vi "Defer Panel Updates.vi"(7 "Set Defer (T)":bool=TRUE, 8 "error in (no error)":errorcluster, 9 "Front Panel (Lookup)":refnum<vi>, 10 "Defer":bool, 11 "Tree (Front Panel)":refnum<vi>) -> (0 "error out":errorcluster, 1 "Front Panel":refnum<vi>)   [LabVIEW 2026, in "Tree Map.lvlib"]
uses:
  Tree Map.lvlib
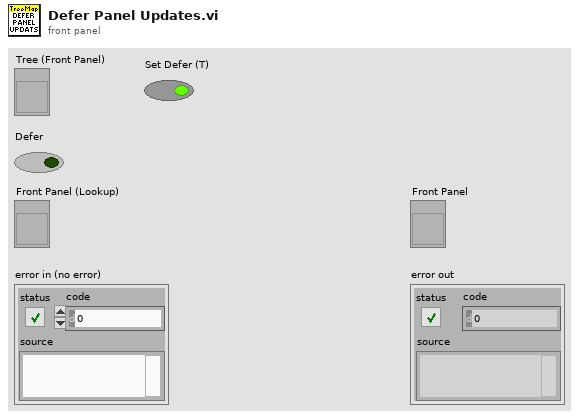
[diagram p1: front panel]
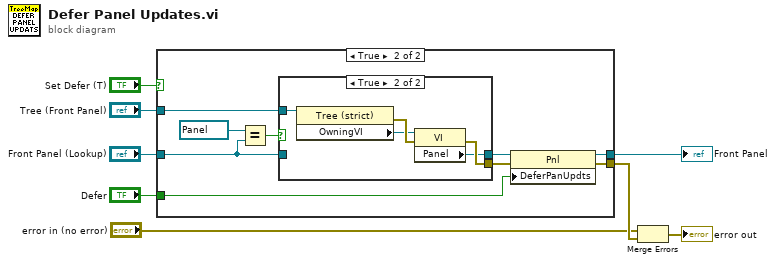
[diagram p0: block diagram]
diagram:
  n1 = case shown="True" "Set Defer (T)" {
    tunnel: "Front Panel (Lookup)" -> [_ w14]
    tunnel: "Defer" -> [_ w13]
    tunnel: [_ w11] -> w6
    tunnel: "Tree (Front Panel)" -> [_ w10]
    tunnel: [_ w9] -> w4
    frame False {
    }
    frame True {
      n2 = Equal?(x=refnum<vi> refnum, y=w14) -> (x = y?=w15:bool)
      n3 = case shown="True" w15 {
        tunnel: [w18 w20] -> w17
        tunnel: w14 -> [w18 _]
        tunnel: [_ w23] -> w12
        tunnel: w10 -> [_ w19]
        frame False {
        }
        frame True {
          n4 = property class="Tree (strict)"(reference=w19) -> (error out=w22:errorcluster, "OwningVI"=w21:refnum<vi>)  [unwired: 1 in, 1 out]
          n5 = property class="VI"(reference=w21, error in=w22) -> (error out=w23:errorcluster, "Panel"=w20:refnum<vi>)  [unwired: 1 out]
        }
      }
      n6 = property class="Pnl"(reference=w17, error in=w12, "DeferPanUpdts"=w13) -> (reference out=w11:refnum<vi>, error out=w9:errorcluster)
    }
  }
  "Front Panel" <- w6
  n7 = Merge Errors("error in (no error)", w4) -> (→"error out":errorcluster)
